vi "DAQmx Reference Trigger (Digital Pattern).vi"(0 "task/channels in":refnum<k21>, 1 "trigger when":i32(ring)=10254 items=["Pattern Matches"=10254, "Pattern Does Not Match"=10253], 5 "source":tag, 7 "pattern":string, 11 "error in":errorcluster, 12 "pretrigger samples per channel":u32=500) -> (4 "task out":refnum<k21>, 15 "error out":errorcluster)   [LabVIEW 2011]
doc: "Configures the task to stop the acquisition when the device acquires all pretrigger samples, matches a digital pattern, and acquires all posttrigger samples. When you use a Reference Trigger, the default for the read RelativeTo property is First PretriggerSample with a read Offset of zero."
uses:
  C:/Program Files/National Instruments/LabVIEW 2011/resource/objmgr/daqmx.rc
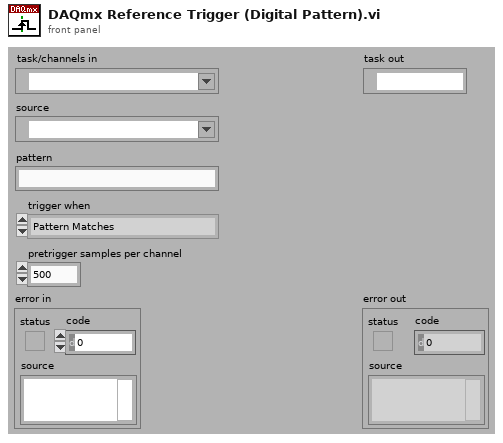
[diagram p1: front panel]
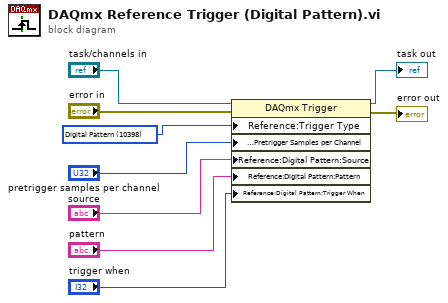
[diagram p0: block diagram]
diagram:
  w5 = 10398 items=["Analog Edge"=10099, "Digital Edge"=10150, "Analog Window"=10103, "Digital Pattern"=10398, "None"=10230] ("Start.TrigType")
  n1 = property class="DAQmx Trigger"(reference="task/channels in", error in="error in", "Reference:Trigger Type"=w5, "Reference:Pretrigger Samples per Channel"="pretrigger samples per channel", "Reference:Digital Pattern:Source"="source", "Reference:Digital Pattern:Pattern"="pattern", "Reference:Digital Pattern:Trigger When"="trigger when") -> (reference out=→"task out":refnum<k21>, error out=→"error out":errorcluster)
